vi "Sample TCP client - LabView 14.vi"() -> ()   [LabVIEW 2022 SP3]
panel:
  out "Parsed reply":T1
  out "JSON Parser error out":errorcluster
  in  "Server port":u16=65432
  in  "Server IP":string="127.0.0.1"
  out "RAW reply":string
  in  "Command input (\"ValidCommand\"\n is the only valid one for this sample)":string="ValidCommand"
  out "TCP error out":errorcluster
  out "Command reply":string
  # "HAHN ROBOTICS BELGIUM"
  # "TCP/IP client + JSON parsing sample code"
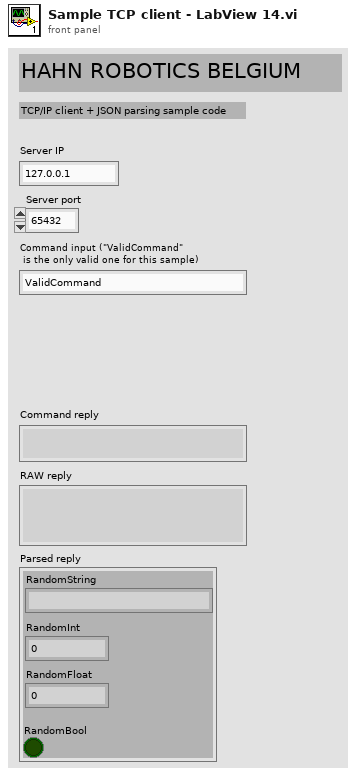
[diagram p1: front panel]
types:
  T1 = cluster{"RandomString":string, "RandomInt":i32, "RandomFloat":dbl, "RandomBool":bool}
  T2 = enum16{"Standard", "Buffered", "CRLF", "Immediate"}
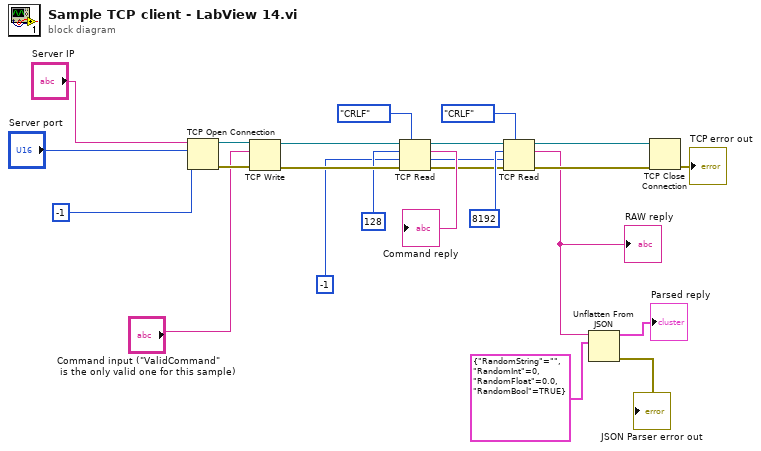
[diagram p0: block diagram]
diagram:
  w1 = -1
  n1 = TCP Open Connection(address="Server IP", remote port or service name="Server port", timeout ms (60000)=-1) -> (connection ID=w21:refnum<k5>, error out=w22:errorcluster)  [unwired: 2 in]
  n2 = TCP Write(connection ID=w21, data in="Command input (\"ValidCommand\"\n is the only valid one for this sample)", error in (no error)=w22) -> (connection ID out=w18:refnum<k5>, error out=w19:errorcluster)  [unwired: 1 in, 1 out]
  n3 = TCP Read(connection ID=w18, bytes to read=128, error in (no error)=w19, 7:T2."CRLF" ("mode (standard)"), 9:w1) -> (connection ID out=w5:refnum<k5>, data out=→"Command reply":string, error out=w6:errorcluster)
  n4 = TCP Read(connection ID=w5, bytes to read=8192, error in (no error)=w6, 7:T2."CRLF" ("mode (standard)"), 9:w1) -> (connection ID out=w14:refnum<k5>, data out=w10:string, error out=w11:errorcluster)
  "RAW reply" <- w10
  n5 = Unflatten From JSON(JSON string=w10, type and defaults=T1 {"RandomString"="", "RandomInt"=0, "RandomFloat"=0.0, "RandomBool"=TRUE}) -> (value=→"Parsed reply":T1, error out=→"JSON Parser error out":errorcluster)  [unwired: 5 in]
  n6 = TCP Close Connection(connection ID=w14, error in (no error)=w11) -> (error out=→"TCP error out":errorcluster)  [unwired: 1 in, 1 out]
